vi "get_config_cluster.vi"(8 "error in (no error)":errorcluster, 11 "GenericPlugin in":refnum<class "LightSourceDL090903Laser.lvclass">) -> (0 "error out":errorcluster, 2 "config cluster (variant)":variant, 3 "GenericPlugin out":refnum<class "LightSourceDL090903Laser.lvclass">)   [LabVIEW 2010, in "LightSourceDL090903Laser.lvclass"]
uses:
  LightSourceDL090903Laser.lvclass
  LightSourceDL090903Laser.lvclass/LightSourceDL090903Laser.ctl
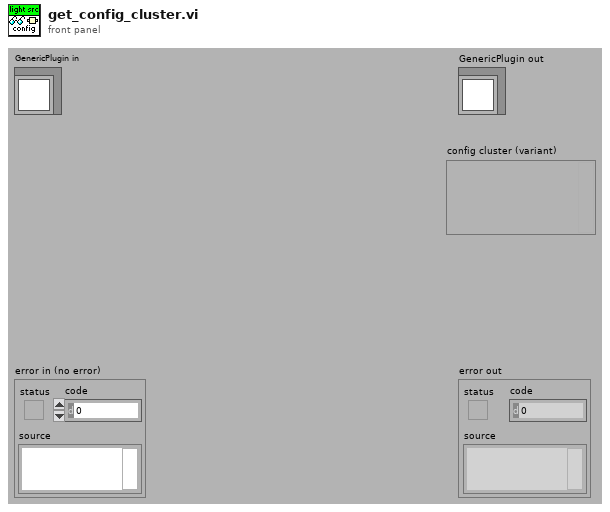
[diagram p1: front panel]
types:
  T1 = typedef "LightSourceDL090903Laser.lvclass/config_data_cluster.ctl" = cluster{"LSID":T2, "manufacturer specification":T3, "type":T4, "laser medium":T5, "frequency multiplication":dbl, "tuneable?":bool, "pulse":T6, "repetition rate":dbl[unit], "pump laser configuration":string}
  T2 = typedef "LSID_cluster.ctl" = cluster{"identifier":string, "revision":i32}
  T3 = typedef "GenericComponent.lvclass/manufacturer_specification_cluster.ctl" = cluster{"manufacturer":string, "model":string, "serial number":string, "lot number":string}
  T4 = typedef "LightSourceDL090903Laser.lvclass/type_enum.ctl" = enum16{"Excimer", "Gas", "MetalVapor", "SolidState", "Dye", "Semiconductor", "FreeElectron", "Unknown"}
  T5 = typedef "LightSourceDL090903Laser.lvclass/laser_medium_enum.ctl" = enum16{"Cu", "Ag", "ArFl", "ArCl", "KrFl", "XeFl", "XeCl", "XeBr", "N", "Ar", "Kr", "Xe", "HeNe", "HeCd", "CO", "CO2", "H2O", "HFl", "NdGlass", "NdYAG", "ErGlass", "ErYAG", "HoYLF", "HoYAG", "Ruby", "TiSapphire", "Alexandrite", "Rhodamine6G", "CoumarineC30", "GaAs", "GaAlAs", "EMinus", "Unknown"}
  T6 = typedef "LightSourceDL090903Laser.lvclass/pulse_enum.ctl" = enum16{"CW", "Single", "QSwitched", "Repetitive", "ModeLocked"}
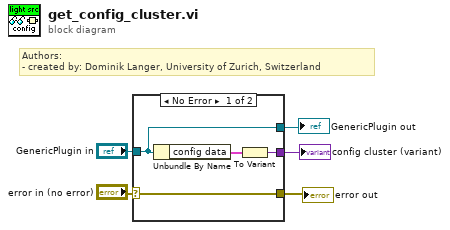
[diagram p0: block diagram]
diagram:
  # "Authors: \n- created by: Dominik Langer, University of Zurich, Switzerland"
  n1 = case shown="No Error" "error in (no error)" {
    selector: "error in (no error)" -> [w6 w10]
    tunnel: "GenericPlugin in" -> [w8 w11]
    tunnel: [w8 w11] -> w3
    tunnel: [w7 _] -> w4
    tunnel: [w6 w10] -> w5
    frame No Error {
      n2 = Unbundle By Name(w8) -> ("config data"=w9:T1)
      n3 = To Variant(anything=w9) -> (Variant=w7:variant)
    }
    frame Error {
    }
  }
  "error out" <- w5
  "GenericPlugin out" <- w3
  "config cluster (variant)" <- w4
